vi "test bench_FXP_Linear_control_law.vi"() -> ()   [LabVIEW 2017]
uses:
  fixed-point/typeDefs/FXPControlParams_distEst.ctl
  fixed-point/typeDefs/x_vec_type.ctl
  fixed-point/typeDefs/UT_matrix_data.ctl
  fixed-point/typeDefs/Bz_vec_scalar.ctl
  fixed-point/typeDefs/Lz_vec_scalar.ctl
  fixed-point/typeDefs/Kz_vec_scalar.ctl
  fixed-point/typeDefs/Nx_vec_scalar.ctl
  fixed-point/typeDefs/Az_vec_scalar.ctl
  fixed-point/typeDefs/x_vec_scalar.ctl
  fixed-point/typeDefs/Cz_vec_scalar.ctl
  fixed-point/typeDefs/x_vec_bram.ctl
  fixed-point/typeDefs/Kz_bram.ctl
  fixed-point/typeDefs/Nx_bram.ctl
  <vilib>/rvi/DataTransferAndStorage/Container/Common/niFpgaContainerExecOnDevCompGetState.vi
  <vilib>/rvi/Emulation/niFpgaEmulationIsFPGAContextNoSignature.vi
  <vilib>/rvi/DataTransferAndStorage/Container/Common/niFpgaContainerGetUniqueNameForEmu.vi
  <vilib>/rvi/Emulation/niFpgaProcessEmulError.vi
  <vilib>/rvi/Emulation/niFpgaSctlEmulationGetInTimedLoop.vi
  <vilib>/rvi/errors/nirviReportUnexpectedCaseInternalError (U32).vi
  <vilib>/rvi/Memory/Memory_Emulation/niFpgaMemoryEmulationCacheClearOnFirstRun.vi
  <vilib>/rvi/Memory/Memory_Emulation/nirvimemoryEmulationManagerCache_MakeExclusive.vi
  <vilib>/rvi/Memory/Memory_Emulation/niFpgaMemoryEmulationValidateCache.vi
  <vilib>/rvi/Memory/Memory_Emulation/nirvimemoryEmulationManagerCache_InsertValue.vi
  <vilib>/Utility/error.llb/Clear Errors.vi
  <vilib>/rvi/Memory/Memory_Emulation/nirvimemoryEmulationManagerCache_ReleaseExclusive.vi
  <vilib>/rvi/Memory/Memory_Emulation/nirvimemoryEmulationManagerCache_GetValue.vi
  <vilib>/rvi/Memory/Memory_Emulation/nirvimemoryEmulationManagerCache_SetValue.vi
  <vilib>/rvi/Emulation/niFpgaSctlEmulationResourceMgr.vi
  <vilib>/rvi/DataTransferAndStorage/Container/XNode/niFpgaContainer.xnode
  <vilib>/rvi/Memory/Memory_Emulation/niFpgaMemoryEmulationRefIn.vi
panel:
  in  "Matrix Data":T1
  out "xerr":T9
  out "xk_12 (out)":T9
  in  "xk_12":T9=[0.0, 0.0, 0.0, 0.0, 0.0, 0.0, 0.0, 0.0, 0.0, 0.0, 0.0, 0.0, 0.0, 0.0, 0.0, 0.0, 0.0, 0.0, 0.0, 0.0, 0.0, 0.0, 0.0, 0.0, 0.0]
  in  "yd_est":fxp<+/-,32,5>
  out "del u(k)":fxp<+/-,64,15>
  out "u_k (saturated)":fxp<+/-,32,5>
  out "saturated?":bool
  in  "ControlParams_distEst":T10={"umax"=3.0, "NS"=0, "ref_f_VEC"=[0.0, 0.0], "Nu11_22"=[0.0, 0.0], "u0"=[0.0, 0.0]} {"ref_f_VEC" format="%#_9g"}
  in  "du_umax":fxp<+/-,18,5>
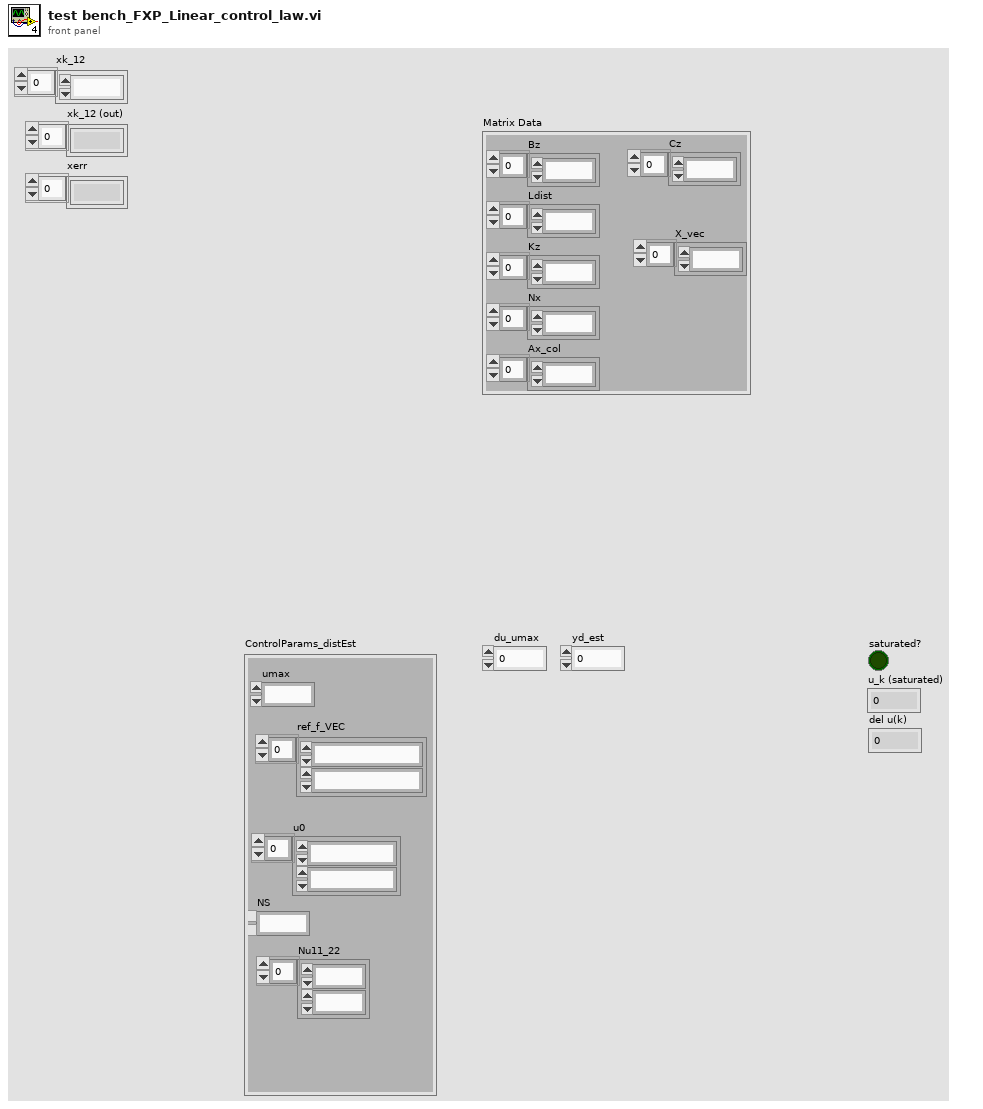
[diagram p1: front panel]
types:
  T1 = typedef "UT_matrix_data.ctl" = cluster{"Bz":T2[], "Ldist":T3[], "Kz":T4[], "Nx":T5[], "Ax_col":T6[], "X_vec":T7[], "Cz":T8[]}
  T2 = typedef "Bz_vec_scalar.ctl" = fxp<+/-,32,3>
  T3 = typedef "Lz_vec_scalar.ctl" = fxp<+/-,32,3>
  T4 = typedef "Kz_vec_scalar.ctl" = fxp<+/-,32,10>
  T5 = typedef "Nx_vec_scalar.ctl" = fxp<+/-,32,2>
  T6 = typedef "Az_vec_scalar.ctl" = fxp<+/-,32,7>
  T7 = typedef "x_vec_scalar.ctl" = fxp<+/-,32,6>
  T8 = typedef "Cz_vec_scalar.ctl" = fxp<+/-,32,4>
  T9 = typedef "x_vec_type.ctl" = fxp<+/-,32,6>[]
  T10 = typedef "FXPControlParams_distEst.ctl" = cluster{"umax":fxp<+/-,18,5>, "NS":u8, "ref_f_VEC":fxp<+/-,32,5>[], "Nu11_22":fxp<+/-,32,5>[], "u0":fxp<+/-,32,5>[]}
  T11 = typedef "x_vec_bram.ctl" = refnum<k21>
  T12 = typedef "Kz_bram.ctl" = refnum<k21>
  T13 = typedef "Nx_bram.ctl" = refnum<k21>
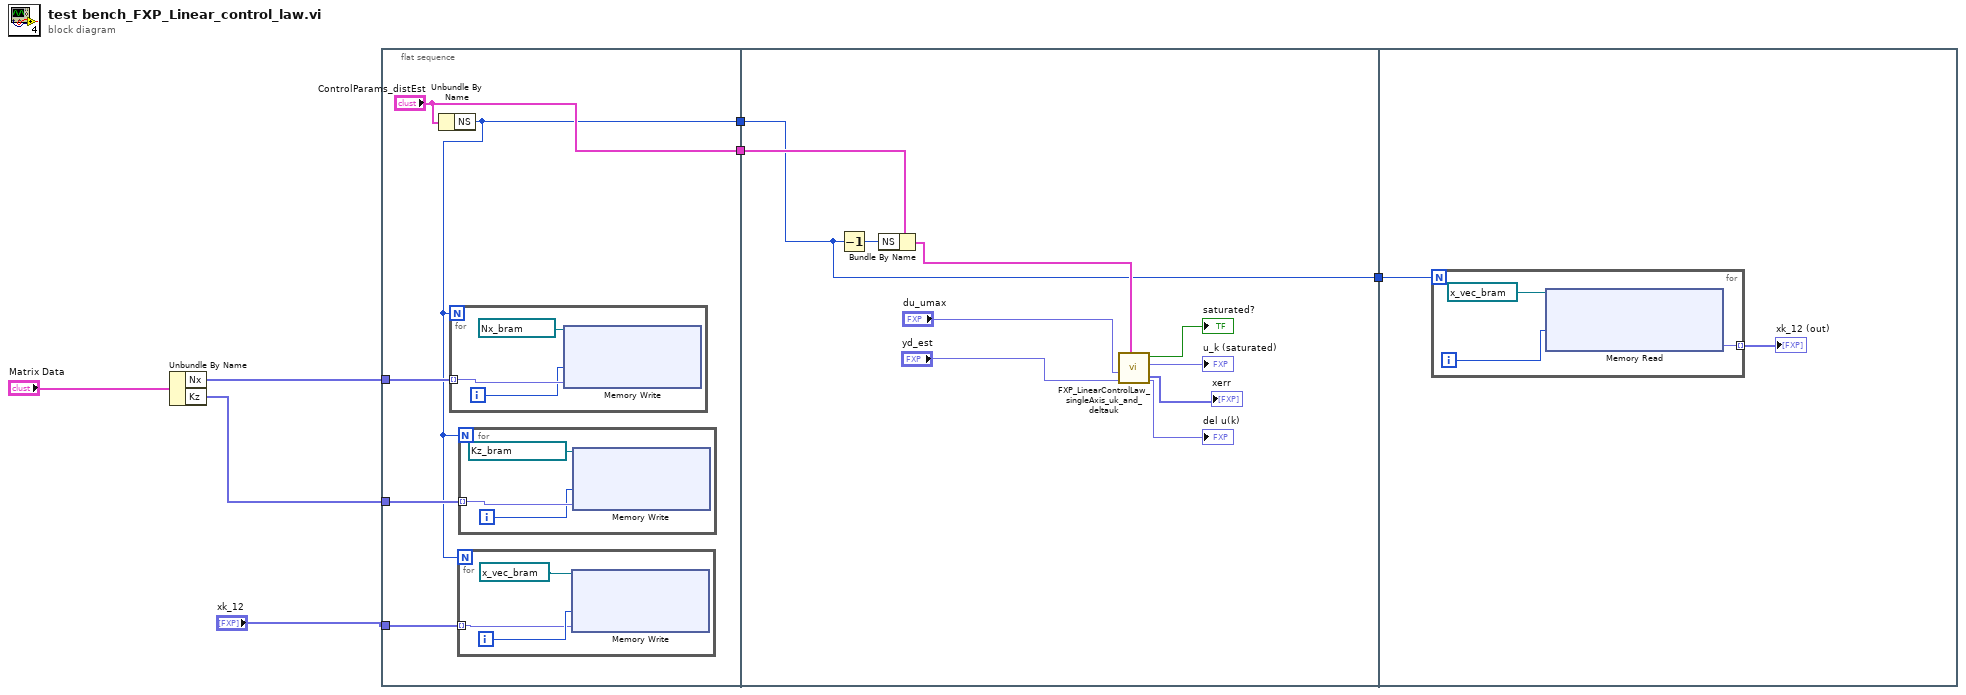
[diagram p0: block diagram]
diagram:
  n1 = Unbundle By Name("Matrix Data") -> ("Nx"=w4:T5[], "Kz"=w3:T4[])
  n2 = flat-sequence {
    tunnel: ["ControlParams_distEst"] -> w6
    tunnel: [w9] -> w5
    tunnel: w4 -> [w11]
    tunnel: w3 -> [w10]
    tunnel: "xk_12" -> [w8]
    tunnel: [w23] -> w7
    tunnel: w6 -> [w31]
    tunnel: w5 -> [w23]
    tunnel: w7 -> [w33]
    frame #0 {
      n3 = Unbundle By Name("ControlParams_distEst") -> ("NS"=w9:u8)
      n4 = for {
        N: w9 -> [_]
        tunnel: w11 -> [w21] mode=indexing
        i -> [w20]
        n5 = xnode "Memory Write"("Address"=w20, "Data"=w21, "Memory In"=T13 "Nx_col1" ("Nx")) -> ()  [unwired: 1 out]
      }
      n6 = for {
        N: w9 -> [_]
        tunnel: w8 -> [w14] mode=indexing
        i -> [w15]
        n7 = xnode "Memory Write"("Address"=w15, "Data"=w14, "Memory In"=T11 "xk_1_2" ("Memory")) -> ()  [unwired: 1 out]
      }
      n8 = for {
        N: w9 -> [_]
        tunnel: w10 -> [w18] mode=indexing
        i -> [w17]
        n9 = xnode "Memory Write"("Address"=w17, "Data"=w18, "Memory In"=T12 "K_FXP_row1" ("Memory")) -> ()  [unwired: 1 out]
      }
    }
    frame #1 {
      n10 = Decrement(x=w23) -> (x-1=w30:u8)
      n11 = Bundle By Name(cluster=w31, "NS"=w30) -> (w24:T10)
      n12 = call "FXP_LinearControlLaw_singleAxis_uk_and_deltauk.vi"("ControlParams_distEst"=w24, "yd_est_x"="yd_est", "du_max"="du_umax") -> ("del u_x"=→"del u(k)":fxp<+/-,64,15>, "u_k (saturated)"=→"u_k (saturated)":fxp<+/-,32,5>, "saturated?"=→"saturated?":bool, "xerr"=→"xerr":fxp<+/-,32,5>[])  [unwired: 5 in]
    }
    frame #2 {
      n13 = for {
        N: w33 -> [_]
        tunnel: [w35] -> w32 mode=indexing
        i -> [w36]
        n14 = xnode "Memory Read"("Address"=w36, "Memory In"=T11 "xk_1_2" ("Memory")) -> ("Data"=w35:fxp<+/-,32,6>)  [unwired: 1 out]
      }
      "xk_12 (out)" <- w32
    }
  }
